vi "UTILITY IP and Computer Name.vi"() -> (2 "IP Address":string, 3 "Computer Name":string)   [LabVIEW 2018]
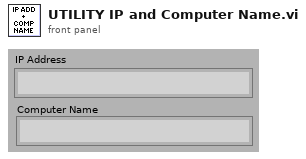
[diagram p1: front panel]
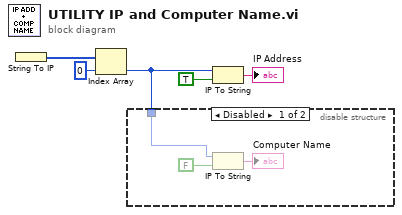
[diagram p0: block diagram]
diagram:
  n1 = String To IP() -> (0:w4:u32[])  [unwired: 1 out]
  n2 = Index Array(array=w4, index=0) -> (element=w1:u32)
  n3 = disable-structure shown="Disabled" {
    disable-tunnel: w1 -> [w6 _]
    frame Disabled {
      n4 = IP To String(1:FALSE ("dot notation? (F)"), 2:w6) -> (0:→"Computer Name":string)
    }
    frame Enabled {
    }
  }
  n5 = IP To String(1:TRUE ("dot notation? (F)"), 2:w1) -> (0:→"IP Address":string)
